vi "MOD.vi"(0 "System no.":i32=1 min=1 max=4 step=1, 2 "ItemID":string[](array[string]), 3 "Value":i32[](array[numeric]), 5 "error in":errorcluster, 6 "Mode ID":i32[](array[numeric])) -> (14 "Controller error":bool, 19 "error out":errorcluster)   [LabVIEW 2020]
doc: "This VI sets modes, waits 100 ms and queries ERR?. See driver manual for available ItemIDs, Mode IDs and values. \n\nE-870: Only one ModeID for only one ItemID per command allowed."
panel:
  # "This vi sets modes, waits 100 ms and queries ERR?.  See driver manual for\navailable ItemIDs, Mode IDs and values."
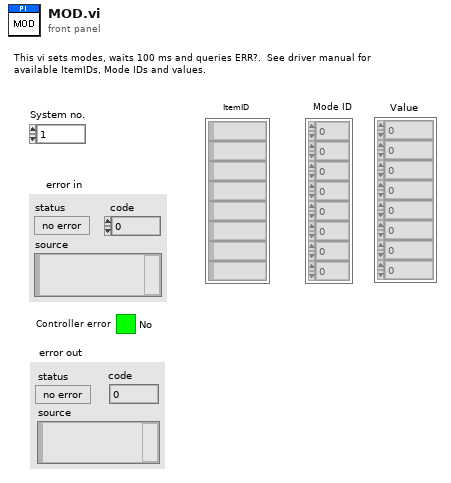
[diagram p1: front panel]
types:
  T1 = enum16{"Disable error check", "Force error check", "Use global settings"}
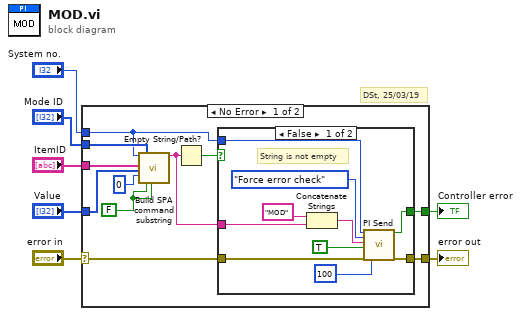
[diagram p0: block diagram]
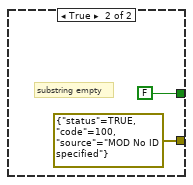
[diagram p2: hidden frame]
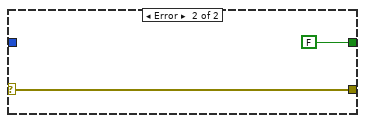
[diagram p3: hidden frame]
diagram:
  # "DSt, 25/03/19"
  n1 = case shown="No Error" "error in" {
    selector: "error in" -> [w10 w31]
    tunnel: [w18 w31] -> w7
    tunnel: "Value" -> [w17 _]
    tunnel: "System no." -> [w14 _]
    tunnel: "ItemID" -> [w16 _]
    tunnel: "Mode ID" -> [w15 _]
    tunnel: [w11 FALSE ("Controller error")] -> w2
    frame No Error {
      w13 = FALSE ("Parameter no. format \n(Decimal: FALSE)")
      n2 = call "Build SPA command substring.vi"("System no."=w14, "Axes to set"=w16, "Parameter values"=w17, "No. of digits"=i16 0 ("No.of digits"), "Parameter number"=w15, "Parameter no. format \n(Decimal: FALSE)"=w13, "Parameter format \n(Num.: FALSE)"=w13) -> ("SPA command substring"=w9:string)  [unwired: 3 in, 9 out]
      n3 = Empty String/Path?(string/path=w9) -> (empty?=w8:bool)
      n4 = case shown="False" w8 {
        tunnel: w9 -> [w27 _]
        tunnel: [w21 errorcluster {"status"=TRUE, "code"=100, "source"="MOD No ID specified"} ("error out")] -> w18
        tunnel: w10 -> [w24 _]
        tunnel: w14 -> [w23 _]
        tunnel: [w20 FALSE ("Controller error")] -> w11
        frame False {
          # "String is not empty"
          n5 = Concatenate Strings("MOD", w27) -> (w25:string)
          n6 = call "PI Send.vi"("System no."=w23, "Error check settings"=T1."Force error check", "String to send"=w25, "Attach termination char.?"=TRUE ("Attach Linefeed?"), "error in"=w24, "Delay before error check (ms)"=u32 100 ("milliseconds to wait")) -> ("Controller error"=w20:bool, "error out"=w21:errorcluster)  [unwired: 12 out]
        }
        frame True {
          # "substring empty"
        }
      }
    }
    frame Error {
    }
  }
  "error out" <- w7
  "Controller error" <- w2
